vi "GE 5565PIORC.Registers.PCIBAR0.Memory Base Address.Set.vi"(8 "error in (no error)":errorcluster, 10 "Memory Base Address":u32, 11 "GE 5565PIORC in":refnum<class "GE 5565PIORC.lvclass">) -> (0 "error out":errorcluster, 3 "GE 5565PIORC out":refnum<class "GE 5565PIORC.lvclass">)   [LabVIEW 2024, in "GE 5565PIORC.lvclass"]
doc: "Memory Base Address for access to Local Configuration registers."
uses:
  GE 5565PIORC.lvclass
  GE 5565PIORC.Registers.PCI Configuration.ctl
  GE 5565PIORC.lvclass/GE 5565PIORC.ctl
  GE 5565PIORC.Registers.PCI Configuration.Read (U32).vi
  GE 5565PIORC.Registers.PCI Configuration.Write (U32).vi
  Methods/GE 5565PIORC.Registers.Read.vi
  Methods/GE 5565PIORC.Registers.Read (U32).vi
  Methods/GE 5565PIORC.Registers.Write.vi
  Methods/GE 5565PIORC.Registers.Write (U32).vi
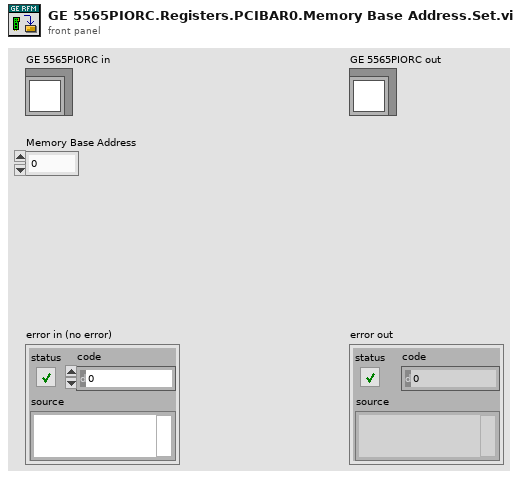
[diagram p1: front panel]
types:
  T1 = typedef "GE 5565PIORC.lvclass/GE 5565PIORC.Registers.PCI Configuration.ctl" = u32
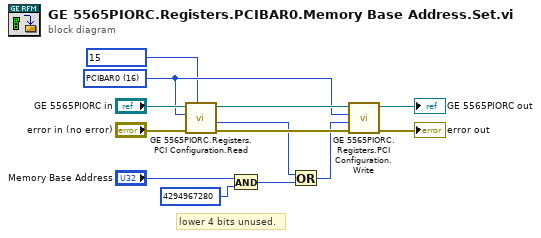
[diagram p0: block diagram]
diagram:
  w5 = T1 16 items=["PCI Configuration ID"=0, "PCI Command"=4, "PCI Status"=6, "PCI Revision ID"=8, "PCI Class Code"=9, "PCI Cache Line Size"=12, "PCI Latency Timer"=13, "PCI Header Type"=14, "PCI Built-in Self Test"=15, "PCIBAR0"=16, "PCIBAR1"=20, "PCIBAR2"=24, "PCIBAR3"=28, "PCIBAR4"=32, "PCIBAR5"=36, "PCI Cardbus CIS Pointer"=40, "PCI Subsystem Vendor ID"=44, "PCI Subsystem ID"=46, "PCI Expansion ROM Base"=48, "Capability Pointer"=52, "PCI Interrupt Line"=60, "PCI Interrupt Pin"=61, "PCI Min_Gnt"=62, "PCI Max_Lat"=63] ("PCI Configuration Registers")
  # "lower 4 bits unused."
  n1 = call-poly "GE 5565PIORC.Registers.PCI Configuration.Read.vi"("Mask (0xFFFFFFFF)"=u32 15, "error in (no error)"="error in (no error)", "Register"=w5, "GE 5565PIORC in"="GE 5565PIORC in") -> ("error out"=w13:errorcluster, "Value"=w4:u32, "GE 5565PIORC out"=w10:refnum<class "GE 5565PIORC.lvclass">)  [unwired: 5 in]
  n2 = And(x="Memory Base Address", y=u32 4294967280 ("Mask (0xFFFFFFFF)")) -> (x .and. y?=w3:u32)
  n3 = Or(x=w4, y=w3) -> (x .or. y?=w2:u32)
  n4 = call-poly "GE 5565PIORC.Registers.PCI Configuration.Write.vi"("error in (no error)"=w13, "Value"=w2, "Register"=w5, "GE 5565PIORC in"=w10) -> ("error out"=→"error out":errorcluster, "GE 5565PIORC out"=→"GE 5565PIORC out":refnum<class "GE 5565PIORC.lvclass">)  [unwired: 6 in]
